vi "Build URL.vi"(8 "error in (no error)":errorcluster, 10 "Value":bool, 11 "HttpButtonControl in":refnum<class "HttpButtonControl.lvclass">) -> (0 "error out":errorcluster, 1 "Post Buffer":string, 2 "URL":string, 3 "HttpButtonControl out":refnum<class "HttpButtonControl.lvclass">)   [LabVIEW 2020, in "VolatusGUIElements.lvlib" / "HttpButtonControl.lvclass"]
uses:
  HttpButtonControl.lvclass
  HttpButtonControl.lvclass/HttpButtonControl.ctl
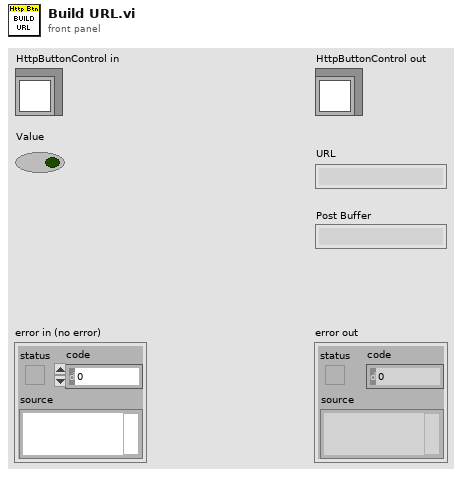
[diagram p1: front panel]
types:
  T1 = typedef "VolatusGUIElements.lvlib/HtmlButtonControl.lvclass/Method.ctl" = enum16{"Get", "Post"}
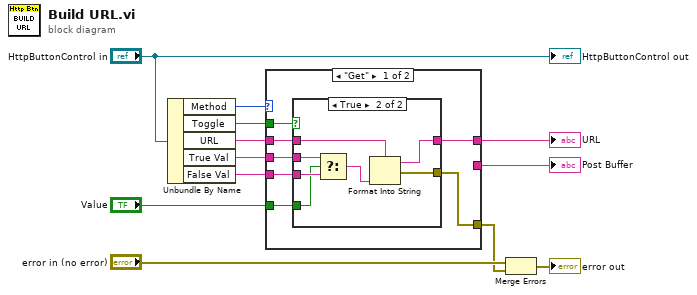
[diagram p0: block diagram]
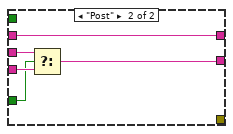
[diagram p3: hidden frame]
diagram:
  n1 = Unbundle By Name("HttpButtonControl in") -> ("Method"=w2:T1, "Toggle"=w10:bool, "URL"=w9:string, "True Val"=w8:string, "False Val"=w7:string)
  n2 = case shown="\"Get\"" w2 {
    tunnel: w10 -> [w19 _]
    tunnel: w9 -> [w18 w32]
    tunnel: w8 -> [w17 w31]
    tunnel: w7 -> [w16 w30]
    tunnel: "Value" -> [w15 w28]
    tunnel: [w14 w32] -> w5
    tunnel: [w13 _] -> w3
    tunnel: [_ w29] -> w1
    frame "Get" {
      n3 = case shown="True" w19 {
        tunnel: w18 -> [w20 w24]
        tunnel: w17 -> [_ w27]
        tunnel: w16 -> [_ w26]
        tunnel: w15 -> [_ w25]
        tunnel: [w20 w22] -> w14
        tunnel: [_ w21] -> w13
        frame False {
        }
        frame True {
          n4 = Select(t=w27, s=w25, f=w26) -> (s? t:f=w23:string)
          n5 = Format Into String(format string=w24, w23) -> (resulting string=w22:string, error out=w21:errorcluster)  [unwired: 2 in]
        }
      }
    }
    frame "Post" {
      n6 = Select(t=w31, s=w28, f=w30) -> (s? t:f=w29:string)
    }
  }
  "URL" <- w5
  "Post Buffer" <- w1
  n7 = Merge Errors("error in (no error)", w3) -> (→"error out":errorcluster)
  "HttpButtonControl out" <- "HttpButtonControl in"
